vi "fgt set sensor Calibration.vi"(8 "error in (no error)":errorcluster, 10 "calibration":T1=enum."H2O", 11 "sensorIndex":u32) -> (0 "error out":errorcluster)   [LabVIEW 2020, in "fgt_SDK.lvlib"]
doc: "Set sensor internal calibration table. Function is only available for IPS (to set new reference value \"zero\") and specific flowrate sensors (dual type) such as the flow-unit M accepting H2O and IPA"
uses:
  fgt_SDK.lvlib
  TypeDefs/fgt_SENSOR_CALIBRATION.ctl
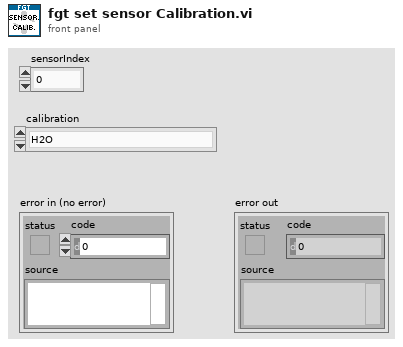
[diagram p1: front panel]
types:
  T1 = typedef "fgt_SDK.lvlib/fgt_SENSOR_CALIBRATION.ctl" = enum16{"None", "H2O", "IPA", "HFE", "FC40", "OIL"}
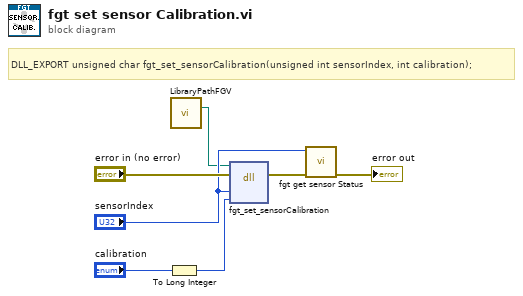
[diagram p0: block diagram]
diagram:
  # "DLL_EXPORT unsigned char fgt_set_sensorCalibration(unsigned int sensorIndex, int calibration);"
  n1 = To Long Integer(number="calibration") -> (32bit integer=w3:i32)
  n2 = call "LibraryPathFGV.vi"() -> ("Path Out"=w1:path)  [unwired: 14 in, 1 out]
  n3 = dll-call lib="C:/Workspace/fgt-SDK/LabVIEW/dlls/fgt_SDK_*.*" fn="fgt_set_sensorCalibration"(path in=w1, error in="error in (no error)", "sensorIndex"="sensorIndex", "calibration"=w3) -> (error out=w5:errorcluster)  [unwired: 4 in, 1 out]
  n4 = call "fgt get sensor Status.vi"("error in (no error)"=w5, "pressureIndex"="sensorIndex") -> ("error out"=→"error out":errorcluster)  [unwired: 9 in]
